vi "Test_Sum_plus_Maj.vi"() -> ()   [LabVIEW 2009]
uses:
  <vilib>/Utility/NIReport.llb/NI_report.lvclass
  <vilib>/Utility/NIReport.llb/HTML/NI_HTML.lvclass
panel:
  in  "Maj (3rd)":bool=TRUE
  out "error out 2":errorcluster
  in  "Sums (4th)":bool=TRUE
  in  "threshold":i32[][](array[numeric])
  out "Instrument VISA out 2":T1={"AWG VISA"="generadorpulsos", "Oscilloscope  VISA "="Oscilloscope", "Integration Board IP"="172.16.7.43", "connection ID"=refnum, "report out"=refnum, "report file path"=path "C:/Documents and Settings/CTA_LAB01/Desktop/L0_Asic/L0 Asic Test Data"}
  in  "IB_Clip":i32[](array[numeric])=[7, 31, 63]
  in  "Adds (2nd)":bool=TRUE
  in  "Sum (1st)":bool=TRUE
  in  "Save NOW!":bool
  in  "Instrument VISA in":T1={"AWG VISA"="generadorpulsos", "Oscilloscope  VISA "="Oscilloscope", "Integration Board IP"="172.16.7.43", "connection ID"=refnum, "report out"=refnum, "report file path"=path "C:/Documents and Settings/CTA_LAB01/Desktop/L0_Asic/L0 Asic Test Data"}
  in  "error in":errorcluster
  in  "Att_gain_b":i32[](array[numeric])=[0, 15]
  in  "Clip_sel":i32[](array[numeric])=[1, 2, 3]
  in  "Channels":i32[](array[numeric])=[0, 1, 2, 3, 4, 5, 6]
  in  "Voltages comprobation":dbl[](array[numeric])=[0.05, 0.1, 0.2, 0.5, 0.8]
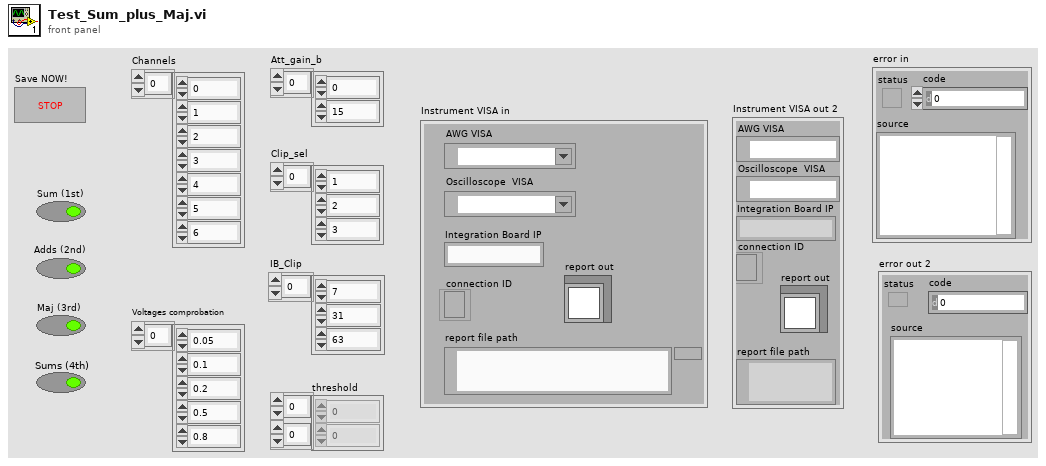
[diagram p1: front panel]
types:
  T1 = cluster{"AWG VISA":refnum<visa-resource-name>, "Oscilloscope  VISA ":refnum<visa-resource-name>, "Integration Board IP":string, "connection ID":refnum<k5>, "report out":refnum<class "NI_report.lvclass">, "report file path":path}
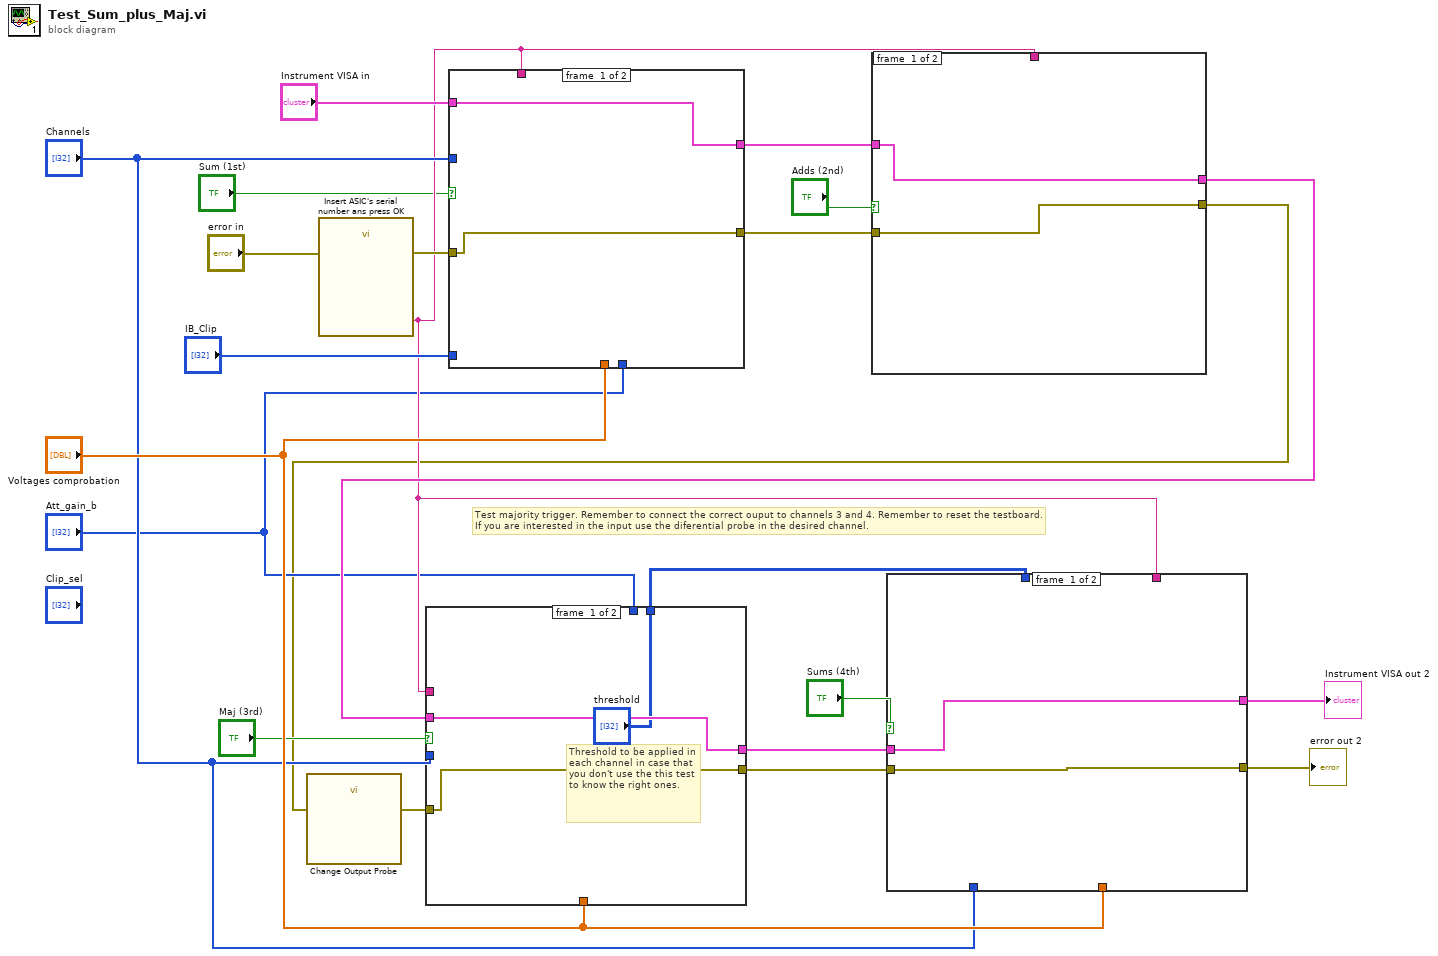
[diagram p0: block diagram]
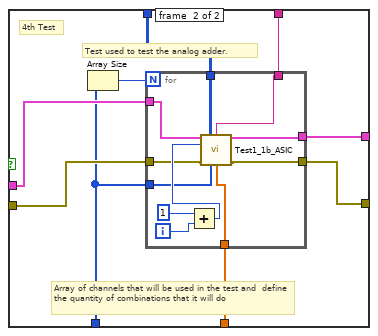
[diagram p2: hidden frame]
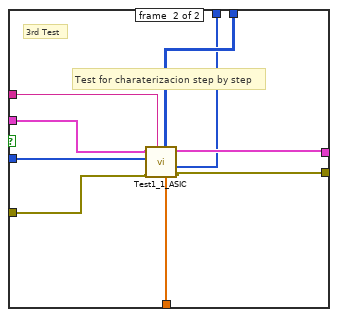
[diagram p3: hidden frame]
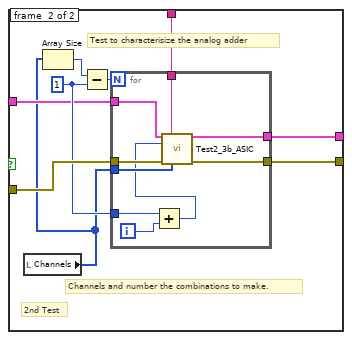
[diagram p4: hidden frame]
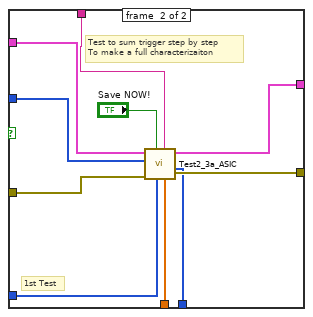
[diagram p5: hidden frame]
diagram:
  # "Test majority trigger. Remember to connect the correct ouput to channels 3 and 4. Remember to reset the testboard. \nIf you are interested in the input use the diferential probe in the desired channel."
  n1 = call "Insert ASIC's serial number ans press OK"("error in (no error)"="error in") -> ("Serial Number"=w5:string, "error out"=w6:errorcluster)  [unwired: 16 in, 1 out]
  n2 = case shown="True" "Sum (1st)" {
    tunnel: "Voltages comprobation" -> [_ w28]
    tunnel: w6 -> [w24 w34]
    tunnel: "Channels" -> [_ w33]
    tunnel: "Instrument VISA in" -> [w23 w32]
    tunnel: "IB_Clip" -> [_ w26]
    tunnel: [w24 w30] -> w21
    tunnel: [w23 w29] -> w20
    tunnel: w5 -> [_ w27]
    tunnel: "Att_gain_b" -> [_ w25]
    frame #0 {
    }
    frame #1 {
      # "1st Test"
      # "Test to sum trigger step by step\nTo make a full characterizaiton"
      n3 = call "Test2_3a_ASIC.vi"("Att. Gain"=w25, "Voltages comprobation"=w28, "Serial number"=w27, "IB_Clip"=w26, "Save NOW!"="Save NOW!", "error in"=w34, "Channels"=w33, "Instrument VISA in"=w32) -> ("error out"=w30:errorcluster, "Instrument VISA out"=w29:T1)  [unwired: 2 in]
    }
  }
  n4 = case shown="True" "Adds (2nd)" {
    tunnel: [w35 w45] -> w11
    tunnel: [w36 w43] -> w1
    tunnel: w21 -> [w36 w44]
    tunnel: w20 -> [w35 w39]
    tunnel: w5 -> [_ w37]
    frame #0 {
    }
    frame #1 {
      w40 = 1 ("y")
      # "2nd Test"
      # "Test to characterisize the analog adder"
      # "Channels and number the combinations to make."
      n5 = local read "Channels"() -> (w38:i32[])
      n6 = Array Size(array=w38) -> (size(s)=w41:i32)
      n7 = Subtract(x=w41, y=w40) -> (x-y=w42:i32)
      n8 = for {
        N: w42 -> [_]
        tunnel: [w54] -> w45
        tunnel: w39 -> [w53]
        tunnel: w44 -> [w52]
        tunnel: [w51] -> w43
        tunnel: w38 -> [w50]
        tunnel: w40 -> [w48]
        tunnel: w37 -> [w46]
        i -> [w49]
        n9 = Add(x=w48, y=w49) -> (x+y=w47:i32)
        n10 = call "Test2_3b_ASIC.vi"("Instrument VISA in"=w53, "Serial Number"=w46, "quantity"=w47, "error in"=w52, "channel array"=w50) -> ("Instrument VISA out"=w54:T1, "error out"=w51:errorcluster)  [unwired: 9 in]
      }
    }
  }
  n11 = call "Change Output Probe"("error in (no error)"=w1) -> ("error out"=w8:errorcluster)  [unwired: 17 in, 1 out]
  n12 = case shown="True" "Maj (3rd)" {
    tunnel: "Voltages comprobation" -> [_ w62]
    tunnel: w8 -> [w57 w64]
    tunnel: "Channels" -> [_ w61]
    tunnel: w11 -> [w56 w63]
    tunnel: [w57 w65] -> w13
    tunnel: [w56 w66] -> w12
    tunnel: ["threshold" w60] -> w14
    tunnel: w5 -> [_ w59]
    tunnel: "Att_gain_b" -> [_ w58]
    frame #0 {
      # "Threshold to be applied in each channel in case that you don't use the this test to know the right ones."
    }
    frame #1 {
      # "3rd Test"
      # "Test for charaterizacion step by step"
      n13 = call "Test1_1_ASIC.vi"("Attenuation"=w58, "Voltages comprobation"=w62, "Serial number"=w59, "error in"=w64, "Channels"=w61, "Instrument VISA in"=w63) -> ("error out"=w65:errorcluster, "Instrument VISA out"=w66:T1, "Array"=w60:i32[][])  [unwired: 3 in]
    }
  }
  n14 = case shown="True" "Sums (4th)" {
    tunnel: [w67 w77] -> w15
    tunnel: [w68 w75] -> w16
    tunnel: w13 -> [w68 w76]
    tunnel: w12 -> [w67 w74]
    tunnel: w14 -> [_ w72]
    tunnel: "Voltages comprobation" -> [_ w71]
    tunnel: "Channels" -> [_ w70]
    tunnel: w5 -> [_ w69]
    frame #0 {
    }
    frame #1 {
      # "4th Test"
      # "Test used to test the analog adder."
      # "Array of channels that will be used in the test and  define the quantity of combinations that it will do"
      n15 = Array Size(array=w70) -> (size(s)=w73:i32)
      n16 = for {
        N: w73 -> [_]
        tunnel: [w87] -> w77
        tunnel: w74 -> [w86]
        tunnel: w76 -> [w84]
        tunnel: [w83] -> w75
        tunnel: w70 -> [w82]
        tunnel: w72 -> [w80]
        tunnel: w71 -> [w79]
        tunnel: w69 -> [w78]
        i -> [w88]
        n17 = Add(x=1 ("y"), y=w88) -> (x+y=w85:i32)
        n18 = call "Test1_1b_ASIC.vi"("Instrument VISA in"=w86, "threshold"=w80, "Serial number"=w78, "quantity"=w85, "error in"=w84, "channel array"=w82, "Voltages comprobation"=w79) -> ("Instrument VISA out"=w87:T1, "error out"=w83:errorcluster)  [unwired: 7 in]
      }
    }
  }
  "Instrument VISA out 2" <- w15
  "error out 2" <- w16
